vi "getPortAndIP.vi"(0 "This Vi":refnum<vi>, 1 "Device Name":string) -> (2 "reference out":refnum<vi>, 3 "port or service name":u16=65400, 4 "Remote Host":string="192.168.10.157")   [LabVIEW 2013]
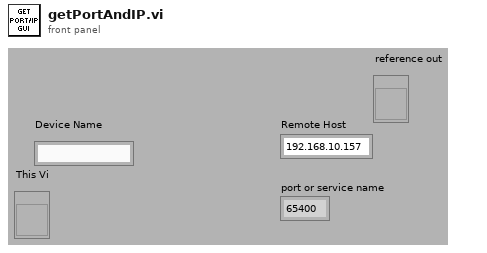
[diagram p1: front panel]
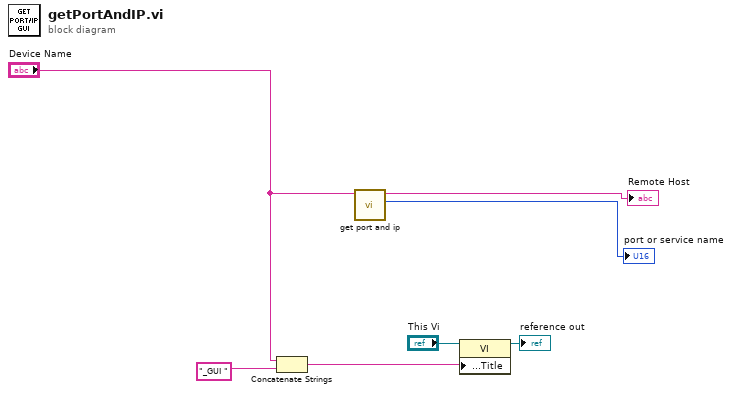
[diagram p0: block diagram]
diagram:
  n1 = Concatenate Strings("Device Name", "_GUI ") -> (w4:string)
  n2 = call "get port and ip.vi"("Device Name"="Device Name") -> ("remote port"=→"port or service name":u16, "remote host ip"=→"Remote Host":string)  [unwired: 7 in, 2 out]
  n3 = property class="VI"(reference="This Vi", "Front Panel.Title"=w4) -> (reference out=→"reference out":refnum<vi>)  [unwired: 1 in, 1 out]
